vi "CMN_GetPhysUnit.vi"(10 "command in":string) -> (1 "unit":string, 2 "command out":string)   [LabVIEW 2016]
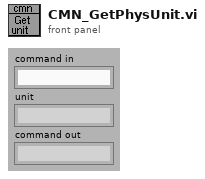
[diagram p1: front panel]
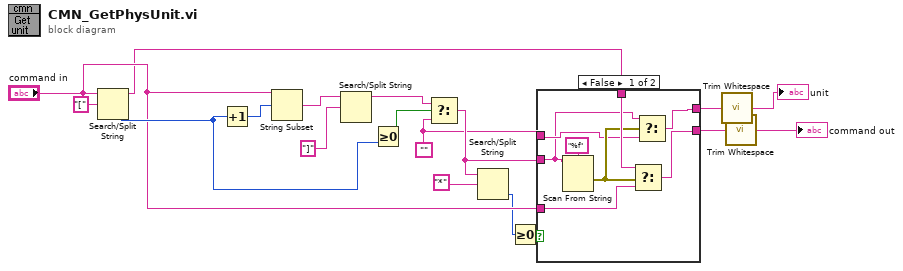
[diagram p0: block diagram]
diagram:
  w4 = ""
  n1 = Search/Split String(string="command in", search string/char (-)="[") -> (substring before match=w9:string, offset of match=w12:i32)  [unwired: 2 out]
  n2 = Increment(x=w12) -> (x+1=w15:i32)
  n3 = String Subset(string="command in", offset (0)=w15) -> (substring=w16:string)  [unwired: 1 out]
  n4 = Search/Split String(string=w16, search string/char (-)="]") -> (substring before match=w13:string)  [unwired: 3 out]
  n5 = Greater Or Equal To 0?(x=w12) -> (x >= 0?=w14:bool)
  n6 = Select(t=w13, s=w14, f=w4) -> (s? t:f=w8:string)
  n7 = Search/Split String(string=w8, search string/char (-)="*") -> (offset of match=w6:i32)  [unwired: 3 out]
  n8 = Greater Or Equal To 0?(x=w6) -> (x >= 0?=w5:bool)
  n9 = case shown="False" w5 {
    tunnel: [w25 w28] -> w11
    tunnel: "command in" -> [w24 w28]
    tunnel: w9 -> [w23 _]
    tunnel: w8 -> [w19 _]
    tunnel: w4 -> [w21 w27]
    tunnel: [w20 w27] -> w3
    frame False {
      n10 = Scan From String(format string="%f", input string=w19) -> (error out=w22:errorcluster)  [unwired: 2 in, 4 out]
      n11 = Select(t=w23, s=w22, f=w24) -> (s? t:f=w25:string)
      n12 = Select(t=w19, s=w22, f=w21) -> (s? t:f=w20:string)
    }
    frame True {
    }
  }
  n13 = call <vilib>:"Trim Whitespace.vi"("string"=w3) -> ("trimmed string"=→"unit":string)  [unwired: 1 in]
  n14 = call <vilib>:"Trim Whitespace.vi"("string"=w11) -> ("trimmed string"=→"command out":string)  [unwired: 1 in]
